vi "Creacion_Tablas_Helice.vi"() -> ()   [LabVIEW 2017]
panel:
  out "Cluster":cluster{"X":dbl, "Y":dbl, "Z":dbl}
  out "Arreglo_Cubo 2":cluster{"X":dbl, "Y":dbl, "Z":dbl}[](array[cluster])=[{"X"=2.0, "Y"=2.0, "Z"=2.0}, {"X"=6.0, "Y"=2.0, "Z"=2.0}, {"X"=6.0, "Y"=6.0, "Z"=2.0}, {"X"=6.0, "Y"=6.0, "Z"=6.0}, {"X"=2.0, "Y"=6.0, "Z"=6.0}, {"X"=2.0, "Y"=2.0, "Z"=6.0}, {"X"=6.0, "Y"=2.0, "Z"=6.0}, {"X"=6.0, "Y"=2.0, "Z"=2.0}, {"X"=6.0, "Y"=6.0, "Z"=2.0}, {"X"=6.0, "Y"=6.0, "Z"=6.0}, {"X"=6.0, "Y"=2.0, "Z"=6.0}, {"X"=6.0, "Y"=2.0, "Z"=2.0}, {"X"=6.0, "Y"=6.0, "Z"=2.0}, {"X"=2.0, "Y"=6.0, "Z"=2.0}, {"X"=2.0, "Y"=6.0, "Z"=6.0}, {"X"=2.0, "Y"=2.0, "Z"=6.0}, {"X"=2.0, "Y"=2.0, "Z"=2.0}, {"X"=2.0, "Y"=6.0, "Z"=2.0}, {"X"=2.0, "Y"=2.0, "Z"=2.0}]
  in  "Desplazamiento Z":dbl=2.0
  in  "Desplazamiento Y":dbl=2.0
  in  "Desplazamiento X":dbl=2.0
  in  "Escala":dbl=4.0
  in  "file path (X)":path=path "C:/Users/LuisFernando/Documents/UPIITA/8vo semestre/Instrumentacion Virtual Aplicada/Solidworks/Sistema_Coordenado_Lectura/Archivos_Lectura/Archivos Cubo/EjeX.txt"
  in  "file path (Z)":path=path "C:/Users/LuisFernando/Documents/UPIITA/8vo semestre/Instrumentacion Virtual Aplicada/Solidworks/Sistema_Coordenado_Lectura/Archivos_Lectura/Archivos Cubo/EjeZ.txt"
  in  "file path (Y)":path=path "C:/Users/LuisFernando/Documents/UPIITA/8vo semestre/Instrumentacion Virtual Aplicada/Solidworks/Sistema_Coordenado_Lectura/Archivos_Lectura/Archivos Cubo/EjeY.txt"
  in  "Arreglo_Cubo":cluster{"X":dbl, "Y":dbl, "Z":dbl}[](array[cluster])=[{"X"=0.0, "Y"=0.0, "Z"=0.0}, {"X"=1.0, "Y"=0.0, "Z"=0.0}, {"X"=1.0, "Y"=1.0, "Z"=0.0}, {"X"=1.0, "Y"=1.0, "Z"=1.0}, {"X"=0.0, "Y"=1.0, "Z"=1.0}, {"X"=0.0, "Y"=0.0, "Z"=1.0}, {"X"=1.0, "Y"=0.0, "Z"=1.0}, {"X"=1.0, "Y"=0.0, "Z"=0.0}, {"X"=1.0, "Y"=1.0, "Z"=0.0}, {"X"=1.0, "Y"=1.0, "Z"=1.0}, {"X"=1.0, "Y"=0.0, "Z"=1.0}, {"X"=1.0, "Y"=0.0, "Z"=0.0}, {"X"=1.0, "Y"=1.0, "Z"=0.0}, {"X"=0.0, "Y"=1.0, "Z"=0.0}, {"X"=0.0, "Y"=1.0, "Z"=1.0}, {"X"=0.0, "Y"=0.0, "Z"=1.0}, {"X"=0.0, "Y"=0.0, "Z"=0.0}, {"X"=0.0, "Y"=1.0, "Z"=0.0}, {"X"=0.0, "Y"=0.0, "Z"=0.0}]
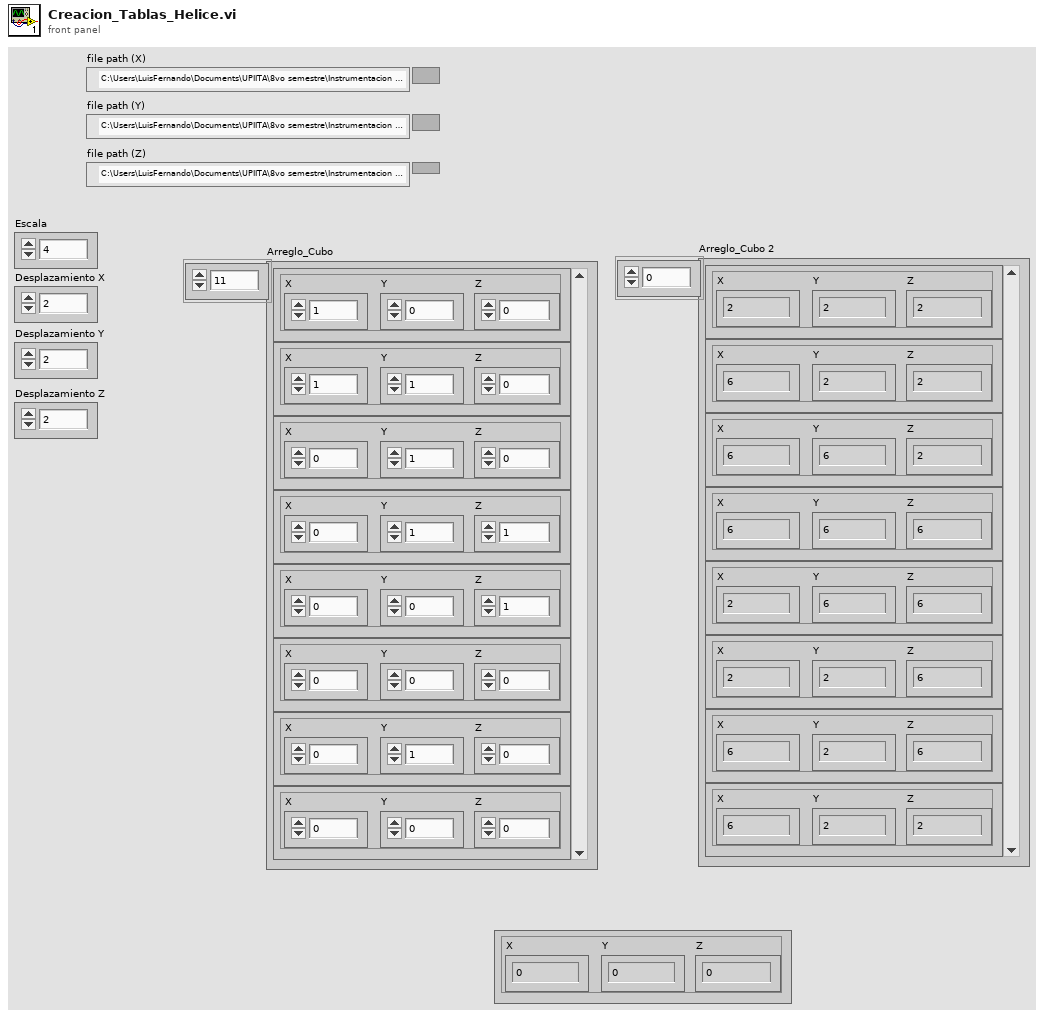
[diagram p1: front panel]
types:
  T1 = enum16{"open", "replace", "create", "open or create", "replace or create", "replace or create with confirmation"}
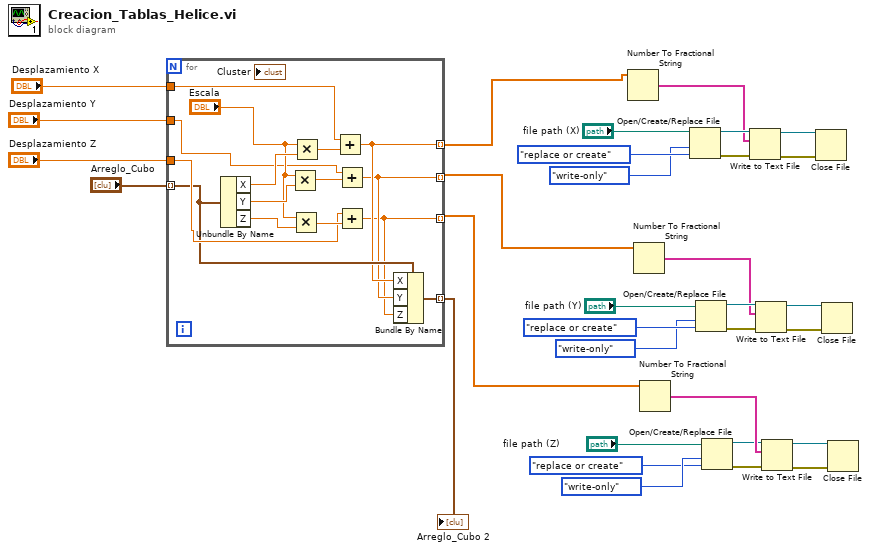
[diagram p0: block diagram]
diagram:
  n1 = for {
    tunnel: "Arreglo_Cubo" -> [w37] mode=indexing
    tunnel: [w36] -> w7 mode=indexing
    tunnel: [w35] -> w6 mode=indexing
    tunnel: [w34] -> w5 mode=indexing
    tunnel: "Desplazamiento X" -> [w40]
    tunnel: "Desplazamiento Y" -> [w38]
    tunnel: "Desplazamiento Z" -> [w39]
    tunnel: [w33] -> w1 mode=indexing
    n2 = Unbundle By Name(w37) -> ("X"=w47:dbl, "Y"=w46:dbl, "Z"=w45:dbl)
    n3 = Multiply(x="Escala", y=w46) -> (x*y=w43:dbl)
    n4 = Multiply(x="Escala", y=w45) -> (x*y=w44:dbl)
    n5 = Multiply(x="Escala", y=w47) -> (x*y=w42:dbl)
    n6 = Add(x=w40, y=w42) -> (x+y=w36:dbl)
    n7 = Add(x=w38, y=w43) -> (x+y=w35:dbl)
    n8 = Add(x=w39, y=w44) -> (x+y=w34:dbl)
    n9 = Bundle By Name(cluster=w37, "X"=w36, "Y"=w35, "Z"=w34) -> (w33:cluster{"X":dbl, "Y":dbl, "Z":dbl})
  }
  "Arreglo_Cubo 2" <- w1
  n10 = Number To Fractional String(number=w7) -> (F-format string=w8:string[])  [unwired: 3 in]
  n11 = Number To Fractional String(number=w6) -> (F-format string=w25:string[])  [unwired: 3 in]
  n12 = Number To Fractional String(number=w5) -> (F-format string=w23:string[])  [unwired: 3 in]
  n13 = Open/Create/Replace File(file path (use dialog)="file path (X)", operation (0:open)=T1."replace or create", access (0:read/write)=enum16{"read/write", "read-only", "write-only"}."write-only") -> (refnum out=w15:refnum<file>, error out=w14:errorcluster)  [unwired: 3 in, 1 out]
  n14 = Open/Create/Replace File(file path (use dialog)="file path (Y)", operation (0:open)=T1."replace or create", access (0:read/write)=enum16{"read/write", "read-only", "write-only"}."write-only") -> (refnum out=w32:refnum<file>, error out=w31:errorcluster)  [unwired: 3 in, 1 out]
  n15 = Open/Create/Replace File(file path (use dialog)="file path (Z)", operation (0:open)=T1."replace or create", access (0:read/write)=enum16{"read/write", "read-only", "write-only"}."write-only") -> (refnum out=w16:refnum<file>, error out=w17:errorcluster)  [unwired: 3 in, 1 out]
  n16 = Write to Text File(file (use dialog)=w15, text=w8, error in=w14) -> (refnum out=w13:refnum<file>, error out=w12:errorcluster)  [unwired: 1 in, 1 out]
  n17 = Write to Text File(file (use dialog)=w32, text=w25, error in=w31) -> (refnum out=w30:refnum<file>, error out=w29:errorcluster)  [unwired: 1 in, 1 out]
  n18 = Write to Text File(file (use dialog)=w16, text=w23, error in=w17) -> (refnum out=w18:refnum<file>, error out=w19:errorcluster)  [unwired: 1 in, 1 out]
  n19 = Close File(refnum=w13, error in=w12) -> ()  [unwired: 2 out]
  n20 = Close File(refnum=w30, error in=w29) -> ()  [unwired: 2 out]
  n21 = Close File(refnum=w18, error in=w19) -> ()  [unwired: 2 out]
